vi "UpdatedImage.vi"(8 "error in (no error)":errorcluster, 10 "Image":T1, 11 "Image Acquisition in":refnum<class "Image Acquisition.lvclass">) -> (0 "error out":errorcluster, 3 "Image Acquisition out":refnum<class "Image Acquisition.lvclass">)   [LabVIEW 2016, in "Image Acquisition.lvlib" / "Image Acquisition.lvclass"]
uses:
  Image Acquisition.lvclass
  <vilib>/vision/Image Controls.llb/IMAQ Image.ctl
  Image Acquisition.lvclass/Image Acquisition.ctl
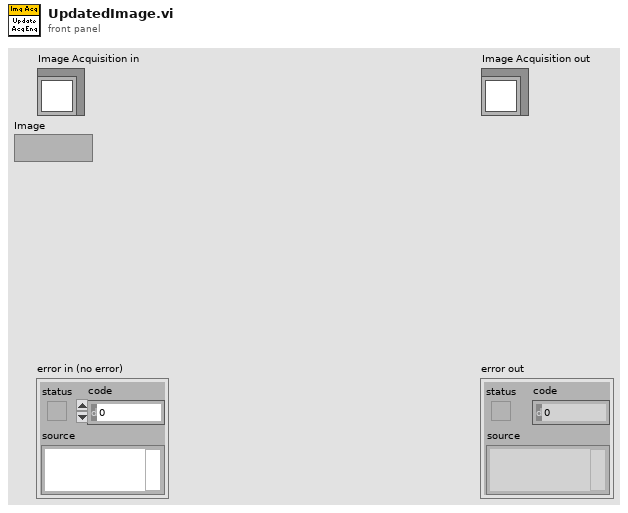
[diagram p1: front panel]
types:
  T1 = typedef "IMAQ Image.ctl" = refnum<image>
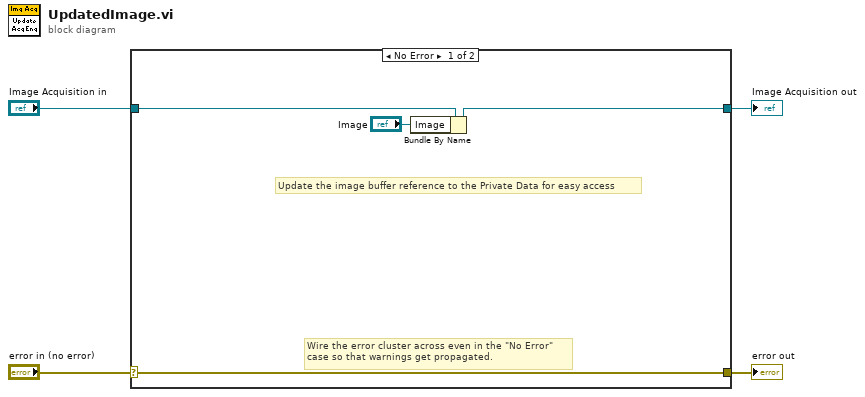
[diagram p0: block diagram]
diagram:
  n1 = case shown="No Error" "error in (no error)" {
    selector: "error in (no error)" -> [w7 w10]
    tunnel: [w7 w10] -> w3
    tunnel: [w6 w9] -> w1
    tunnel: "Image Acquisition in" -> [w8 w9]
    frame No Error {
      # "Update the image buffer reference to the Private Data for easy access"
      # "Wire the error cluster across even in the \"No Error\"\ncase so that warnings get propagated."
      n2 = Bundle By Name(cluster=w8, "Image"="Image") -> (w6:refnum<class "Image Acquisition.lvclass">)
    }
    frame Error {
    }
  }
  "error out" <- w3
  "Image Acquisition out" <- w1
